vi "LCR Example.vi"() -> ()   [LabVIEW 2018]
uses:
  controls/LCR function.ctl
  <instrlib>/BK Precision 891/BK Precision 891.lvlib
panel:
  out "Measured Secondary Reading":dbl
  out "Measured Primary Reading":dbl
  in  "VISA resource name":refnum<visa-resource-name>
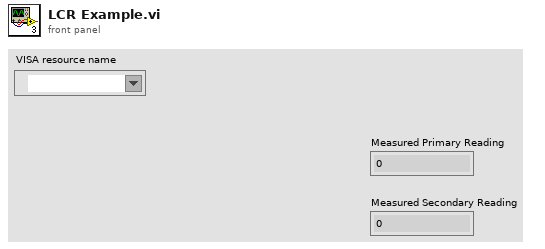
[diagram p1: front panel]
types:
  T1 = typedef "LCR function.ctl" = u16
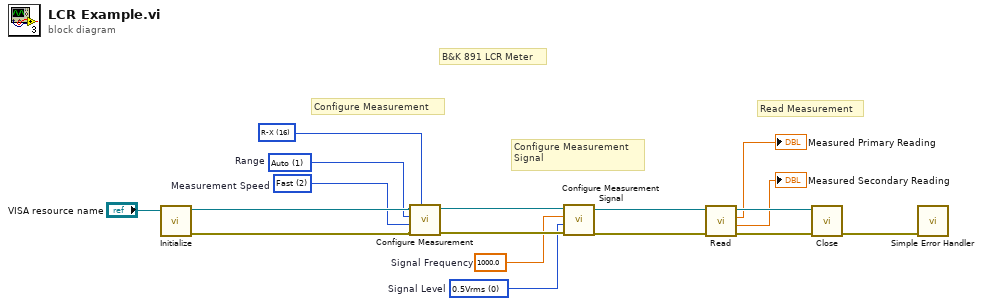
[diagram p0: block diagram]
diagram:
  w1 = T1 16 items=["Cs-Q", "Cs-D", "Cs-R", "Cp-Q", "Cp-D", "Cp-R", "Cp-G", "Ls-Q", "Ls-D", "Ls-R", "Lp-Q", "Lp-D", "Lp-R", "Lp-G", "Z-th", "Y-th", "R-X", "G-B", "DCR"] ("Function (4: Cp-D)")
  w2 = u8 0 items=["0.5Vrms", "1Vrms"]  # Signal Level
  w3 = 1000.0  # Signal Frequency
  w6 = u16 2 items=["Slow"=1, "Fast"=2]  # Measurement Speed
  w7 = u16 1 items=["Hold", "Auto"]  # Range
  # "Configure Measurement\nSignal"
  # "Read Measurement"
  # "Configure Measurement"
  # "B&K 891 LCR Meter"
  n1 = call <instrlib>:"Initialize.vi"("VISA resource name"="VISA resource name") -> ("error out"=w8:errorcluster, "VISA resource name out"=w9:refnum<visa-resource-name>)  [unwired: 9 in]
  n2 = call <instrlib>:"Configure Measurement.vi"("Function (4: Cp-D)"=w1, "error in (no error)"=w8, "Measurement Speed (2:Fast)"=w6, "Range (1:Auto)"=w7, "VISA resource name"=w9) -> ("error out"=w10:errorcluster, "VISA resource name out"=w11:refnum<visa-resource-name>)  [unwired: 5 in]
  n3 = call <instrlib>:"Configure Measurement Signal.vi"("error in (no error)"=w10, "Signal Level (0:0.5 Vrms)"=w2, "Signal Frequency (1000 Hz)"=w3, "VISA resource name"=w11) -> ("error out"=w4:errorcluster, "VISA resource name out"=w5:refnum<visa-resource-name>)  [unwired: 6 in]
  n4 = call <instrlib>:"Read.vi"("error in (no error)"=w4, "VISA resource name"=w5) -> ("error out"=w15:errorcluster, "Measured Secondary Reading"=→"Measured Secondary Reading":dbl, "Measured Primary Reading"=→"Measured Primary Reading":dbl, "VISA resource name out"=w16:refnum<visa-resource-name>)  [unwired: 6 in]
  n5 = call <instrlib>:"Close.vi"("error in (no error)"=w15, "VISA resource name"=w16) -> ("error out"=w12:errorcluster)  [unwired: 9 in]
  n6 = call <vilib>:"Simple Error Handler.vi"("error in (no error)"=w12) -> ()  [unwired: 4 in, 5 out]
